vi "Stop.vi"(8 "error in (no error)":errorcluster, 11 "Process In":refnum<class "Debug View.lvclass">) -> (0 "error out":errorcluster, 3 "Process Out":refnum<class "Debug View.lvclass">)   [LabVIEW 2020, in "Debug View.lvclass"]
doc: "Sends a stop message to the process, which must perform a safe shut down. This VI waits for the process to call the Finish method or times out if the configured time out expires. If the method does not time out, the process returned by this VI contains the full state of the process when it was stopped."
uses:
  Debug View.lvclass
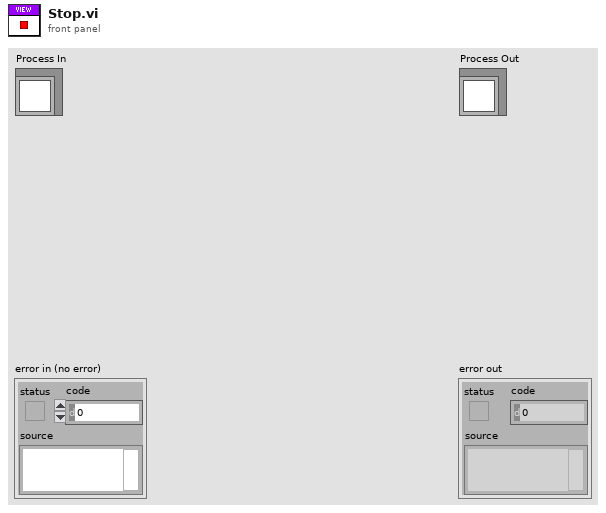
[diagram p1: front panel]
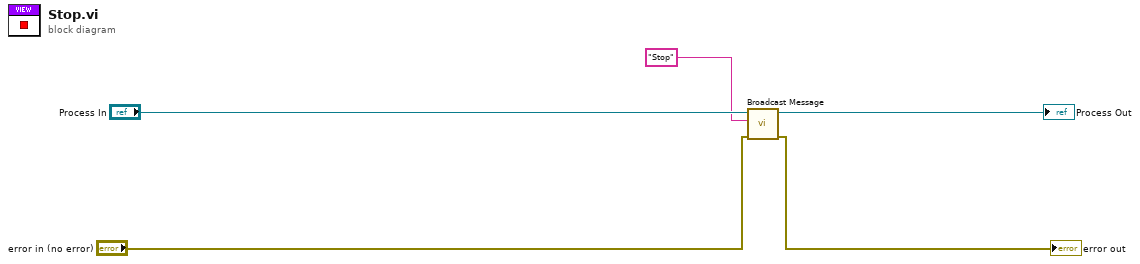
[diagram p0: block diagram]
diagram:
  n1 = call-dynamic "Broadcast Message.vi"("error in (no error)"="error in (no error)", "Message"="Stop", "Debug View In"="Process In") -> ("error out"=→"error out":errorcluster, "Debug View Out"=→"Process Out":refnum<class "Debug View.lvclass">)  [unwired: 7 in]
